vi "Elevator Manual Control 3.0.vi"(9 "Down":bool, 10 "Up":bool, 11 "Enabled":bool) -> (3 "Motor Output":dbl)   [LabVIEW 2014]
panel:
  out "Down in range":bool
  out "Up In range":bool
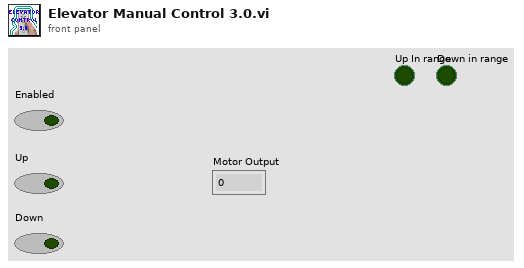
[diagram p1: front panel]
types:
  T1 = typedef "WPI_PotentiometerDevRef.ctl" = cluster{"DevStatus":errorcluster, "Controller":T2, "Analog Channel":T3, "Invert Output":bool}
  T2 = typedef "FPGA_TypedefAnalogModule.ctl" = enum16{"Controller 1"}
  T3 = typedef "FPGA_AIChannel.ctl" = enum8{"AI 0", "AI 1", "AI 2", "AI 3", "AI MXP 0", "AI MXP 1", "AI MXP 2", "AI MXP 3", "Invalid"}
  T4 = typedef "WPI_MotorControlDeviceRef.ctl" = cluster{"DeviceStatus":errorcluster, "Type":T5, "PWM":cluster{"Controller":T6, "PWM Channel":T7, "DeadBand":T8}, "CAN":cluster{"Device Number":u8, "Control Mode":T9, "Semaphore":T10, "Max Vout":dbl, "TalonSRX Control Mode":T11}, "Invert":bool, "TransformRef":T12, "InvTransformRef":T12}
  T5 = typedef "WPI_MotorControlType.ctl" = enum16{"PWM", "CAN", "CANTalonSRX"}
  T6 = typedef "FPGA_TypedefDigitalModule.ctl" = enum16{"Controller 1"}
  T7 = typedef "FPGA_DIOPWMChannel.ctl" = enum8{"PWM 0", "PWM 1", "PWM 2", "PWM 3", "PWM 4", "PWM 5", "PWM 6", "PWM 7", "PWM 8", "PWM 9", "PWM MXP 0", "PWM MXP 1", "PWM MXP 2", "PWM MXP 3", "PWM MXP 4", "PWM MXP 5", "PWM MXP 6", "PWM MXP 7", "PWM MXP 8", "PWM MXP 9", "Invalid"}
  T8 = typedef "WPI_PWMDeadband.ctl" = cluster{"Name":string, "maxPositivePwm":i32, "minPositivePwm":i32, "centerPwm":i32, "maxNegativePwm":i32, "minNegativePwm":i32, "angularRange":u16}
  T9 = typedef "WPI_CANJaguar_ControlMode.ctl" = enum8{"Percent VBus", "Current", "Speed", "Position", "Voltage"}
  T10 = typedef "Semaphore RefNum" = refnum<k1>
  T11 = typedef "WPI_CANTalonSRX_APIControlMode.ctl" = enum8{"Percent VBus", "Speed", "Position", "Slave", "Unchanged / Invalid"}
  T12 = typedef "WPI_PWMTransform_ConPane.ctl" = refnum<vi>
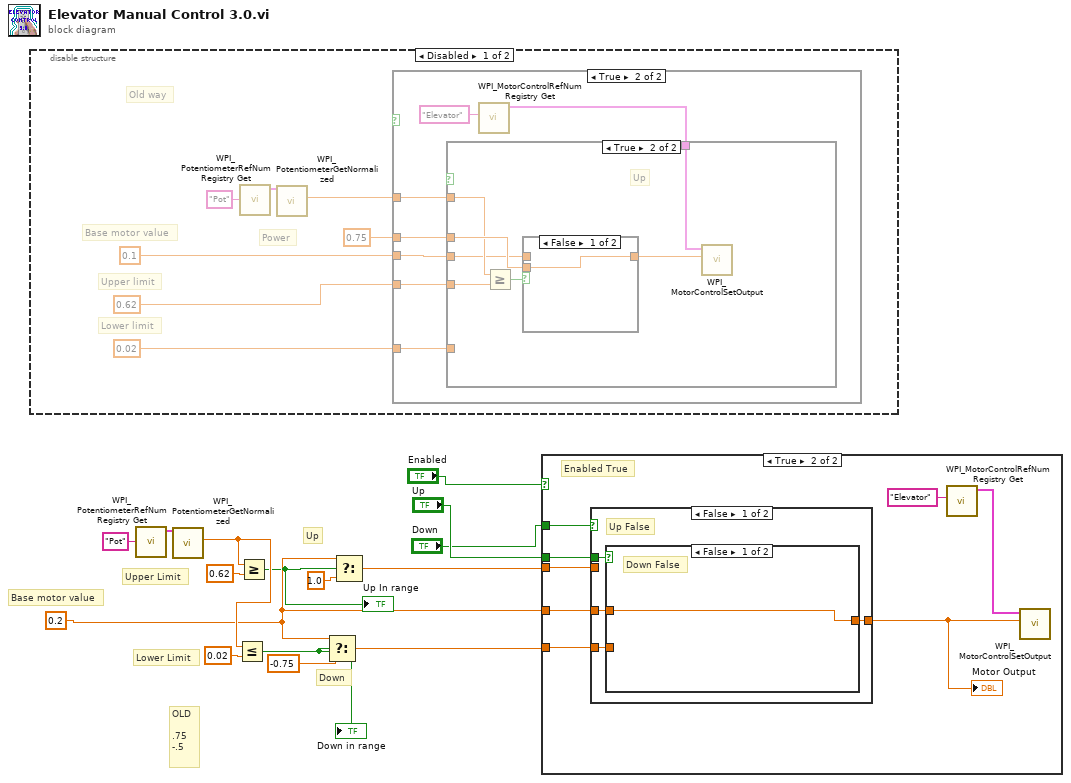
[diagram p0: block diagram]
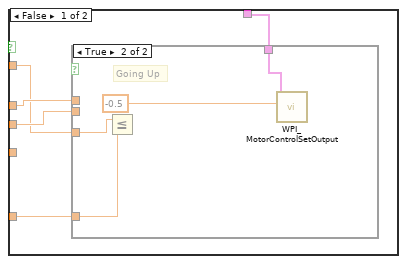
[diagram p3: hidden frame]
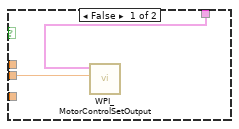
[diagram p4: hidden frame]
diagram:
  w7 = 0.2 ("Output")
  # "OLD \n\n.75\n-.5"
  # "Base motor value"
  # "Down"
  # "Up"
  # "Lower Limit"
  # "Upper Limit"
  n1 = disable-structure shown="Disabled" {
    frame Disabled {
      # "Old way"
      # "Power"
      # "Lower limit"
      # "Upper limit"
      # "Base motor value"
      n2 = call <vilib>:"WPI_PotentiometerRefNum Registry Get.vi"("refnum name"="Pot") -> ("PotDevRef"=w16:T1)  [unwired: 9 in, 1 out]
      n3 = call <vilib>:"WPI_PotentiometerGetNormalized.vi"("PotDevRef"=w16) -> ("Normalized Value"=w19:dbl)  [unwired: 8 in, 2 out]
      n4 = case shown="True" {
        selector: _ -> [_ _]
        tunnel: 0.1 ("Output") -> [_ w27]
        tunnel: 0.75 ("Output") -> [_ w26]
        tunnel: w19 -> [_ w25]
        tunnel: 0.62 ("Output") -> [_ w24]
        tunnel: 0.02 ("Output") -> [_ w23]
        frame False {
        }
        frame True {
          n5 = call <vilib>:"WPI_MotorControlRefNum Registry Get.vi"("refnum name"="Elevator") -> ("MotorControlDevRef"=w29:T4)  [unwired: 9 in, 1 out]
          n6 = case shown="True" {
            selector: _ -> [_ _]
            tunnel: w29 -> [w34 w47]
            tunnel: w27 -> [w33 w41]
            tunnel: w26 -> [w32 w45]
            tunnel: w25 -> [w31 w43]
            tunnel: w24 -> [_ w42]
            tunnel: w23 -> [w30 _]
            frame False {
              n7 = case shown="True" {
                selector: _ -> [_ _]
                tunnel: w34 -> [w36 w40]
                tunnel: w33 -> [w35 _]
                tunnel: w32 -> [_ _]
                tunnel: w31 -> [_ w39]
                tunnel: w30 -> [_ w38]
                frame False {
                  n8 = call <vilib>:"WPI_MotorControlSetOutput.vi"("Output"=w35, "MotorControlDevRef"=w36) -> ()  [unwired: 7 in, 3 out]
                }
                frame True {
                  # "Going Up"
                  n9 = Less Or Equal?(x=w39, y=w38) -> ()  [unwired: 1 out]
                  n10 = call <vilib>:"WPI_MotorControlSetOutput.vi"("Output"=-0.5, "MotorControlDevRef"=w40) -> ()  [unwired: 7 in, 3 out]
                }
              }
            }
            frame True {
              # "Up"
              n11 = Greater Or Equal?(x=w43, y=w42) -> (x >= y?=w44:bool)
              n12 = case shown="False" w44 {
                tunnel: [w48 w49] -> w46
                tunnel: w45 -> [w48 _]
                tunnel: w41 -> [_ w49]
                frame False {
                }
                frame True {
                }
              }
              n13 = call <vilib>:"WPI_MotorControlSetOutput.vi"("Output"=w46, "MotorControlDevRef"=w47) -> ()  [unwired: 7 in, 3 out]
            }
          }
        }
      }
    }
    frame Enabled {
    }
  }
  n14 = call <vilib>:"WPI_PotentiometerRefNum Registry Get.vi"("refnum name"="Pot") -> ("PotDevRef"=w14:T1)  [unwired: 9 in, 1 out]
  n15 = call <vilib>:"WPI_PotentiometerGetNormalized.vi"("PotDevRef"=w14) -> ("Normalized Value"=w12:dbl)  [unwired: 8 in, 2 out]
  n16 = Less Or Equal?(x=w12, y=0.02) -> (x <= y?=w10:bool)
  "Down in range" <- w10
  n17 = Greater Or Equal?(x=w12, y=0.62) -> (x >= y?=w3:bool)
  "Up In range" <- w3
  n18 = Select(t=w7, s=w10, f=-0.75) -> (s? t:f=w6:dbl)
  n19 = Select(t=w7, s=w3, f=1.0) -> (s? t:f=w5:dbl)
  n20 = case shown="True" "Enabled" {
    tunnel: w7 -> [_ w54]
    tunnel: w6 -> [_ w53]
    tunnel: w5 -> [_ w52]
    tunnel: "Down" -> [_ w51]
    tunnel: "Up" -> [_ w50]
    frame False {
      # "Manual control is disabled"
    }
    frame True {
      # "Enabled True"
      n21 = case shown="False" w51 {
        tunnel: [w61 w64] -> w55
        tunnel: w54 -> [w60 _]
        tunnel: w53 -> [w59 _]
        tunnel: w52 -> [_ w64]
        tunnel: w50 -> [w58 _]
        frame False {
          # "Up False"
          n22 = case shown="False" w58 {
            tunnel: [w62 w63] -> w61
            tunnel: w60 -> [w62 _]
            tunnel: w59 -> [_ w63]
            frame False {
              # "Down False"
            }
            frame True {
              # "Down True"
            }
          }
        }
        frame True {
          # "Up True"
        }
      }
      "Motor Output" <- w55
      n23 = call <vilib>:"WPI_MotorControlRefNum Registry Get.vi"("refnum name"="Elevator") -> ("MotorControlDevRef"=w57:T4)  [unwired: 9 in, 1 out]
      n24 = call <vilib>:"WPI_MotorControlSetOutput.vi"("Output"=w55, "MotorControlDevRef"=w57) -> ()  [unwired: 7 in, 3 out]
    }
  }
